vi "Load Octree.vi"(0 "Octree file path":path) -> (1 "Octree node array":T1[](array[typedef]), 2 "Error out":errorcluster)   [LabVIEW 2014]
uses:
  Typedefs/TreeNodeBox.ctl
  Typedefs/Quad.ctl
  Typedefs/Quadplane enum.ctl
panel:
  # "PN 23/01/2015"
  # "Vertices"
  # "Edges"
  # "Unit normal"
  # "Plane ident."
  # "Vertices"
  # "Edges"
  # "Unit normal"
  # "Plane ident."
  # "Vertices"
  # "Edges"
  # "Unit normal"
  # "Plane ident."
  # "Vertices"
  # "Edges"
  # "Unit normal"
  # "Plane ident."
  # "Vertices"
  # "Edges"
  # "Unit normal"
  # "Plane ident."
  # "Vertices"
  # "Edges"
  # "Unit normal"
  # "Plane ident."
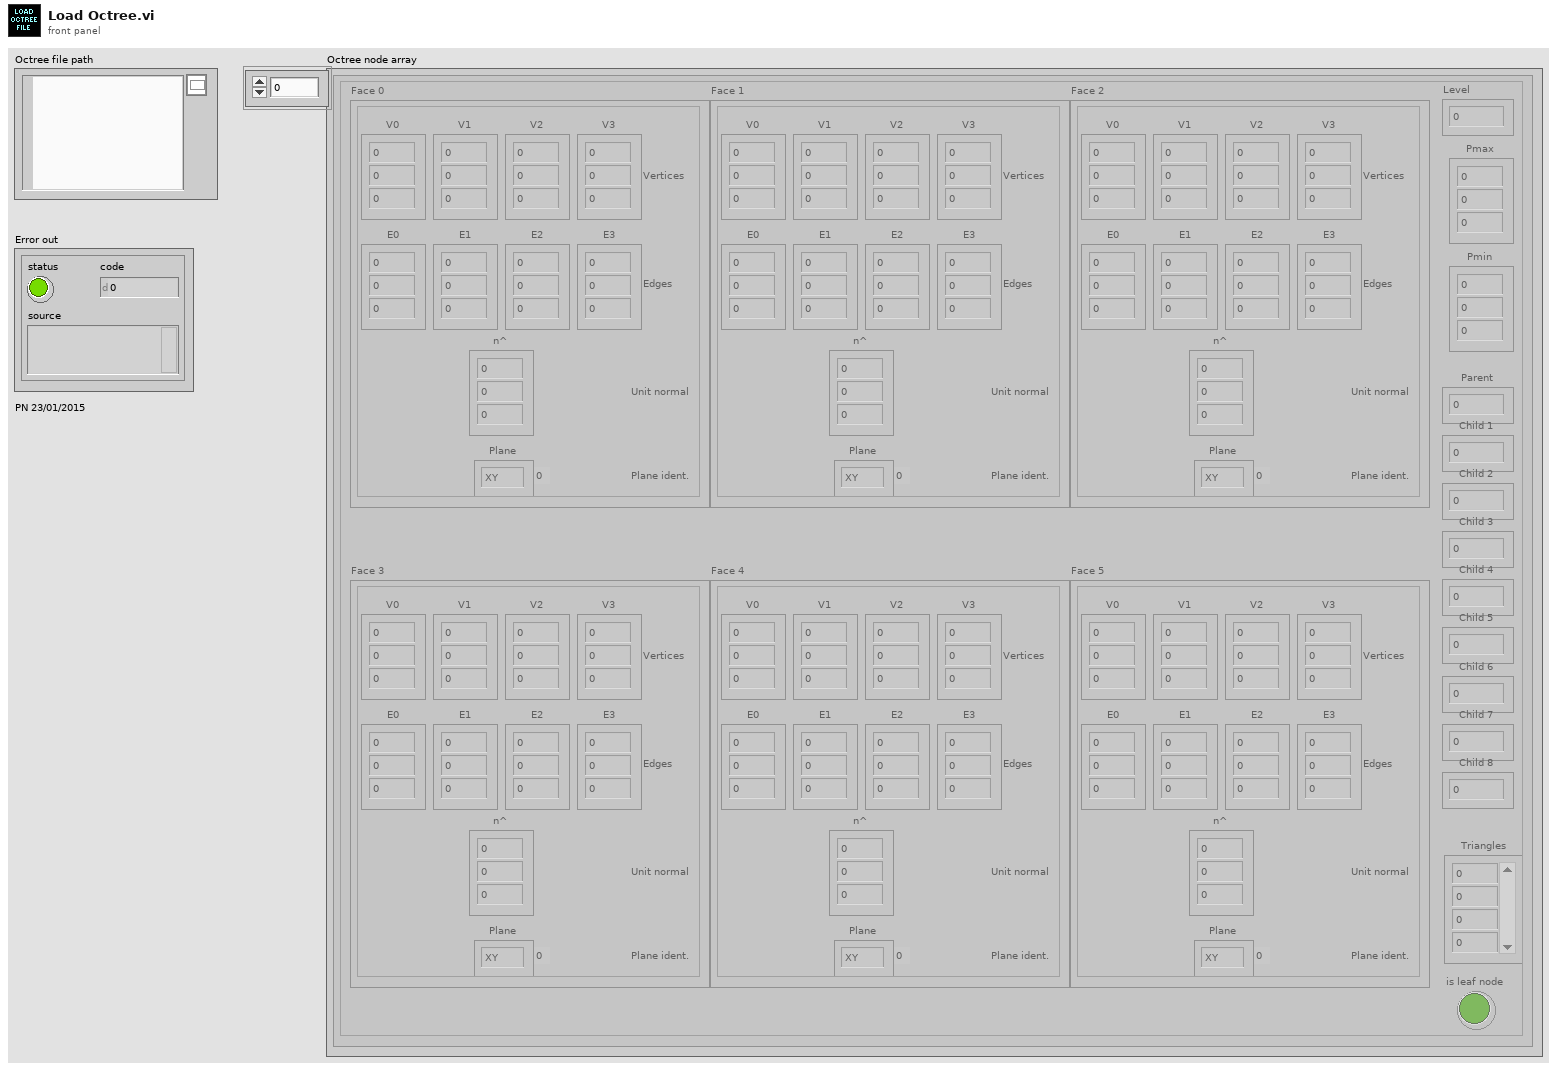
[diagram p1: front panel]
types:
  T1 = typedef "TreeNodeBox.ctl" = cluster{"Face 0":T2, "Face 1":T2, "Face 2":T2, "Face 3":T2, "Face 4":T2, "Face 5":T2, "Level":i32, "Pmax":sgl[], "Pmin":sgl[], "Parent":i32, "Child 1":i32, "Child 2":i32, "Child 3":i32, "Child 4":i32, "Child 5":i32, "Child 6":i32, "Child 7":i32, "Child 8":i32, "Triangles":i32[], "is leaf node":bool}
  T2 = typedef "Quad.ctl" = cluster{"V0":sgl[], "V1":sgl[], "V2":sgl[], "V3":sgl[], "E0":sgl[], "E1":sgl[], "E2":sgl[], "E3":sgl[], "n^":sgl[], "Plane":T3}
  T3 = typedef "Quadplane enum.ctl" = enum8{"XY", "XZ", "YZ", "-XY", "-XZ", "-YZ"}
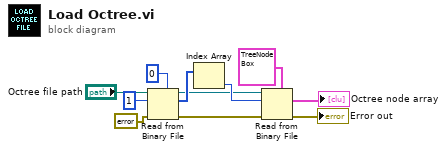
[diagram p0: block diagram]
diagram:
  n1 = Read from Binary File(5:0 ("count (1)"), 8:errorcluster {"status"=FALSE, "code"=0, "source"=""} ("error in (no error)"), 10:1 ("count (1)"), 11:"Octree file path") -> (0:w9:errorcluster, 2:w6:i32[], 3:w4:refnum<file>)  [unwired: 2 in, 1 out]
  n2 = Index Array(array=w6) -> (element=w5:i32)  [unwired: 1 in]
  n3 = Read from Binary File(5:T1 {"Face 0"={"V0"=[], "V1"=[], "V2"=[], "V3"=[], "E0"=[], "E1"=[], "E2"=[], "E3"=[], "n^"=[], "Plane"=enum."XY"}, "Face 1"={"V0"=[], "V1"=[], "V2"=[], "V3"=[], "E0"=[], "E1"=[], "E2"=[], "E3"=[], "n^"=[], "Plane"=enum."XY"}, "Face 2"={"V0"=[], "V1"=[], "V2"=[], "V3"=[], "E0"=[], "E1"=[], "E2"=[], "E3"=[], "n^"=[], "Plane"=enum."XY"}, "Face 3"={"V0"=[], "V1"=[], "V2"=[], "V3"=[], "E0"=[], "E1"=[], "E2"=[], "E3"=[], "n^"=[], "Plane"=enum."XY"}, "Face 4"={"V0"=[], "V1"=[], "V2"=[], "V3"=[], "E0"=[], "E1"=[], "E2"=[], "E3"=[], "n^"=[], "Plane"=enum."XY"}, "Face 5"={"V0"=[], "V1"=[], "V2"=[], "V3"=[], "E0"=[], "E1"=[], "E2"=[], "E3"=[], "n^"=[], "Plane"=enum."XY"}, "Level"=0, "Pmax"=[], "Pmin"=[], "Parent"=0, "Child 1"=0, "Child 2"=0, "Child 3"=0, "Child 4"=0, "Child 5"=0, "Child 6"=0, "Child 7"=0, "Child 8"=0, "Triangles"=[], "is leaf node"=FALSE} ("Box"), 8:w9, 10:w5, 11:w4) -> (0:→"Error out":errorcluster, 2:→"Octree node array":T1[])  [unwired: 2 in, 2 out]
